vi "IMAQController.UpdateCameraList.vi"(1 "activatedCameras":T2(array[cluster]), 4 "Detector.ini List Camera-Array":string[](array[string])) -> (15 "actItem Number":i32[](array[numeric]), 18 "Item Names":string[][](array[string]))   [LabVIEW 2014, in "IMAQController.lvlib"]
uses:
  IMAQController.lvlib
  <vilib>/Utility/miscctls.llb/LVPoint32TypeDef.ctl
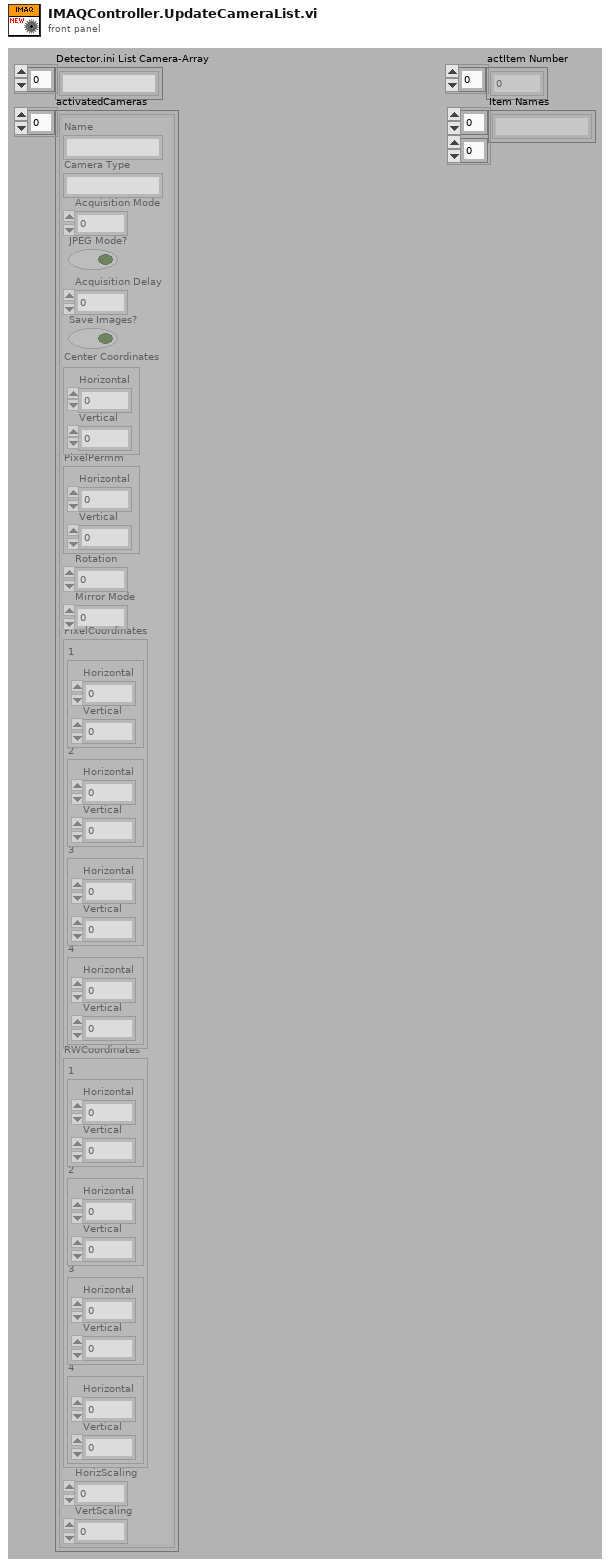
[diagram p1: front panel]
types:
  T1 = typedef "LVPoint32TypeDef.ctl" = cluster{"Horizontal":i32, "Vertical":i32}
  T2 = cluster{"Name":string, "Camera Type":string, "Acquisition Mode":u32, "JPEG Mode?":bool, "Acquisition Delay":dbl, "Save Images?":bool, "Center Coordinates":T1, "PixelPermm":cluster{"Horizontal":dbl, "Vertical":dbl}, "Rotation":dbl, "Mirror Mode":u32, "PixelCoordinates":cluster{"1":cluster{"Horizontal":i32, "Vertical":i32}, "2":cluster{"Horizontal":i32, "Vertical":i32}, "3":cluster{"Horizontal":i32, "Vertical":i32}, "4":cluster{"Horizontal":i32, "Vertical":i32}}, "RWCoordinates":cluster{"1":cluster{"Horizontal":dbl, "Vertical":dbl}, "2":cluster{"Horizontal":dbl, "Vertical":dbl}, "3":cluster{"Horizontal":dbl, "Vertical":dbl}, "4":cluster{"Horizontal":dbl, "Vertical":dbl}}, "HorizScaling":dbl, "VertScaling":dbl}[]
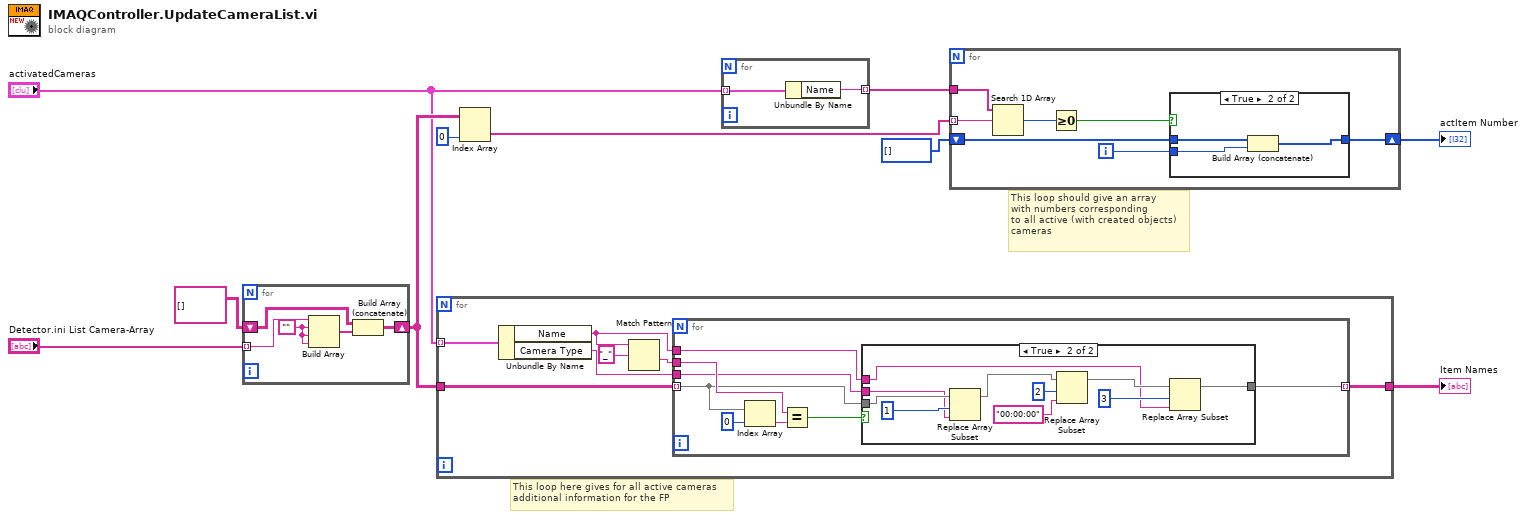
[diagram p0: block diagram]
diagram:
  # "This loop here gives for all active cameras\nadditional information for the FP"
  # "This loop should give an array\nwith numbers corresponding\nto all active (with created objects)\ncameras"
  n1 = for {
    tunnel: "Detector.ini List Camera-Array" -> [w11] mode=indexing
    shift-right: [w14] -> w8
    shift-left: string[][] [] ("Item Names") -> [w15]
    w12 = ""
    n2 = Build Array(w11, w12, w12, w12) -> (w13:string[])
    n3 = Build Array (concatenate)(w15, w13) -> (w14:string[][])
  }
  n4 = for {
    tunnel: "activatedCameras" -> [w22] mode=indexing
    tunnel: w8 -> [w20]
    tunnel: [w17] -> w9
    n5 = Unbundle By Name(w22) -> ("Name"=w16:string, "Camera Type"=w18:string)
    n6 = Match Pattern(string=w16, regular expression="_") -> (after substring=w19:string)  [unwired: 1 in, 3 out]
    n7 = for {
      tunnel: w20 -> [w26] mode=indexing
      tunnel: w19 -> [w30]
      tunnel: [w25] -> w17 mode=indexing
      tunnel: w18 -> [w24]
      tunnel: w16 -> [w23]
      n8 = Index Array(array=w26, index=0) -> (element=w29:string)
      n9 = Equal?(x=w30, y=w29) -> (x = y?=w27:bool)
      n10 = case shown="True" w27 {
        tunnel: w26 -> [w31 w41]
        tunnel: [w31 w34] -> w25
        tunnel: w24 -> [_ w36]
        tunnel: w23 -> [_ w32]
        frame False {
        }
        frame True {
          n11 = Replace Array Subset(array=w41, new element=w36, index=1) -> (w40:string[])
          n12 = Replace Array Subset(array=w40, new element="00:00:00" ("new element/subarray"), index=2) -> (w35:string[])
          n13 = Replace Array Subset(array=w35, new element=w32, index=3) -> (w34:string[])
        }
      }
    }
  }
  "Item Names" <- w9
  n14 = Index Array(array=w8, index (col)=0 ("disabled index (col)")) -> (element=w6:string[])  [unwired: 1 in]
  n15 = for {
    tunnel: "activatedCameras" -> [w43] mode=indexing
    tunnel: [w42] -> w5 mode=indexing
    n16 = Unbundle By Name(w43) -> ("Name"=w42:string)
  }
  n17 = for {
    tunnel: w6 -> [w49] mode=indexing
    tunnel: w5 -> [w50]
    shift-right: [w44] -> w3
    shift-left: i32[] [] ("actCameras 2") -> [w45]
    i -> [w46]
    n18 = Search 1D Array(1D array=w50, element=w49) -> (index of element=w48:i32)  [unwired: 1 in]
    n19 = Greater Or Equal To 0?(x=w48) -> (x >= 0?=w47:bool)
    n20 = case shown="True" w47 {
      tunnel: w46 -> [_ w52]
      tunnel: w45 -> [w51 w54]
      tunnel: [w51 w53] -> w44
      frame False {
      }
      frame True {
        n21 = Build Array (concatenate)(w54, w52) -> (w53:i32[])
      }
    }
  }
  "actItem Number" <- w3
